vi "PXIe-5172_Init.vi"(8 "Error In":errorcluster, 11 "Object in":refnum<class "PXIe-5172.lvclass">=refnum) -> (0 "Error Out":errorcluster, 3 "object out":refnum<class "PXIe-5172.lvclass">)   [LabVIEW 2023, in "PXIe-5172.lvlib" / "PXIe-5172.lvclass"]
uses:
  PXIe-5172.lvclass
panel:
  in  "HW Device Name":string
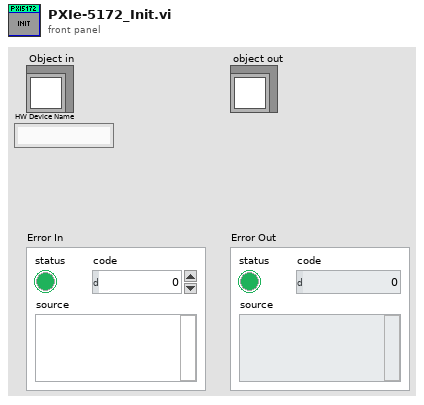
[diagram p1: front panel]
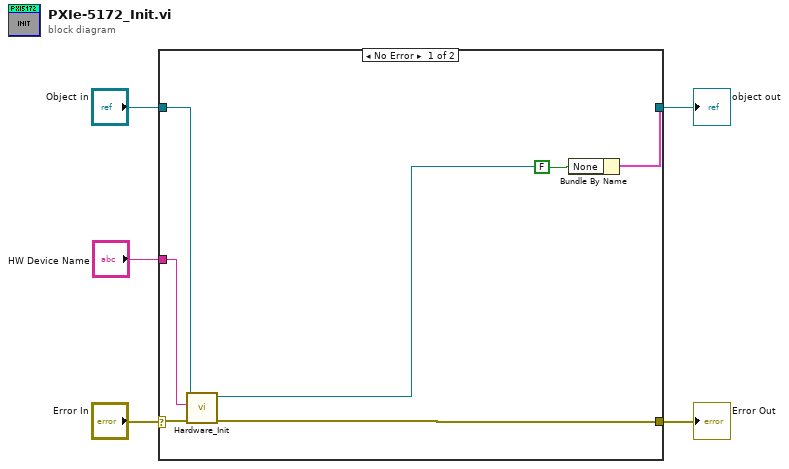
[diagram p0: block diagram]
diagram:
  n1 = case shown="No Error" "Error In" {
    selector: "Error In" -> [w10 w13]
    tunnel: [w12 w14] -> w5
    tunnel: "Object in" -> [w8 w14]
    tunnel: [w9 w13] -> w2
    tunnel: "HW Device Name" -> [w6 _]
    frame No Error {
      n2 = call "Hardware_Init.vi"("Error In"=w10, 10:w6, "object in"=w8) -> ("Error Out"=w9:errorcluster, "object in"=w7:refnum<class "PXIe-5172.lvclass">)  [unwired: 7 in]
      n3 = Bundle By Name(cluster=w7, "None"=FALSE) -> (w12:cluster{})
    }
    frame Error {
    }
  }
  "object out" <- w5
  "Error Out" <- w2
